vi "Test Run Suite of Several Suites.vi"(8 "error in (no error)":errorcluster, 11 "Test Case In":refnum<class "LUnit Test Suite Tests.lvclass">) -> (0 "error out":errorcluster, 3 "Test Case Out":refnum<class "LUnit Test Suite Tests.lvclass">)   [LabVIEW 2020, in "LUnit Test Suite Tests.lvclass"]
uses:
  LUnit Test Suite Tests.lvclass
  C:/Program Files (x86)/National Instruments/LabVIEW 2020/vi.lib/Astemes/LUnit/Test Case.lvclass
  source/API/LUnit Test Suite/LUnit Test Suite.lvclass
  C:/git/astemes-lunit/source/Core/Runnable/Runnable.lvclass
  Test Case Test Double/Test Case Test Double.lvclass
  C:/git/astemes-lunit/source/Core/LUnit Test Case/LUnit Test Case.lvclass
  <vilib>/Astemes/LUnit/Test Case.lvclass/Test Case.ctl
  b74e4934-f044-4222-b3dd-fc90e6c1bd4f.vi
  <vilib>/Astemes/LUnit/Palette/Pass.vi
  <vilib>/Astemes/LUnit/Palette/Fail.vi
  <vilib>/Astemes/LUnit/Compare Variants.vi
  <vilib>/Astemes/LUnit/Describe Comparison.vi
  <vilib>/Astemes/LUnit/Set Assertion Type.vi
  <vilib>/Astemes/LUnit/Add test result.vi
  <vilib>/Astemes/LUnit/Variant to string.vi
  <vilib>/Astemes/LUnit/LUnit Record Assertion Result.vi
  <vilib>/Astemes/LUnit/LUnit Aggregate Assertion Results.vi
  <vilib>/Astemes/LUnit/Method Result/LUnit Merge Status.vi
  <vilib>/Astemes/LUnit/LUnit Concatenate result strings.vi
  <vilib>/Utility/Data Type/Get Type Information.vi
  <vilib>/Utility/LVClass/Get LV Class Name.vi
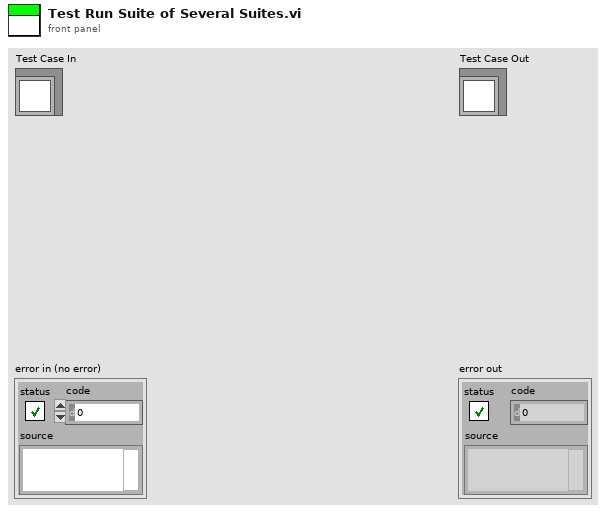
[diagram p1: front panel]
types:
  T1 = typedef "Result.lvlib/Result.ctl" = cluster{"Name":string, "Message":string, "Description":string, "Status":T2, "Result Type":T3, "Execution Time":dbl}
  T2 = typedef "Result.lvlib/Status.ctl" = enum16{"", "Passed", "Failed", "Error", "Skipped", "Setup Error", "Broken", "Teardown Error"}
  T3 = typedef "Result.lvlib/Type.ctl" = enum16{"Method", "Case", "Suite", "Pass", "Fail", "Skip", "Pass if", "Fail if", "Pass if Error", "Fail if Error", "Pass if Equal", "Fail if Equal"}
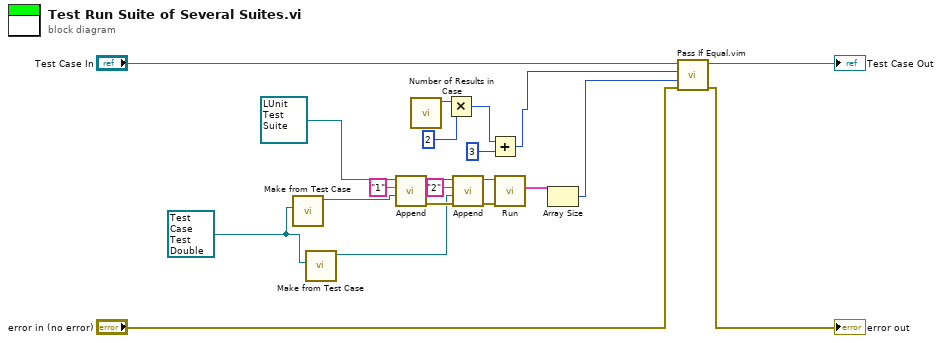
[diagram p0: block diagram]
diagram:
  w10 = refnum<class "Test Case Test Double.lvclass"> refnum ("LUnit Test Case V2 out")
  n1 = call "Make from Test Case.vi"("LUnit Test Case"=w10) -> ("LUnit Test Suite Out"=w9:refnum<class "LUnit Test Suite.lvclass">)  [unwired: 9 in, 1 out]
  n2 = call "Make from Test Case.vi"("LUnit Test Case"=w10) -> ("LUnit Test Suite Out"=w8:refnum<class "LUnit Test Suite.lvclass">)  [unwired: 9 in, 1 out]
  n3 = call "Append.vi"("Runnable"=w9, "Name"="1", "LUnit Test Suite In"=refnum<class "LUnit Test Suite.lvclass"> refnum ("LUnit Test Suite V2 in")) -> ("error out"=w13:errorcluster, "LUnit Test Suite Out"=w12:refnum<class "LUnit Test Suite.lvclass">)  [unwired: 7 in]
  n4 = call "Number of Results in Case.vi"() -> ("Number of Results"=w4:i32)  [unwired: 11 in]
  n5 = Multiply(x=w4, y=2) -> (x*y=w2:i32)
  n6 = call "Append.vi"("error in (no error)"=w13, "Runnable"=w8, "Name"="2", "LUnit Test Suite In"=w12) -> ("error out"=w15:errorcluster, "LUnit Test Suite Out"=w14:refnum<class "LUnit Test Suite.lvclass">)  [unwired: 6 in]
  n7 = Add(x=w2, y=3 ("size(s)")) -> (x+y=w3:i32)
  n8 = call-dynamic "Run.vi"("error in (no error)"=w15, "LUnit Test Suite In"=w14) -> ("Results"=w17:T1[])  [unwired: 8 in, 1 out]
  n9 = Array Size(array=w17) -> (size(s)=w16:i32)
  n10 = call "Pass If Equal.vim"("error in (no error)"="error in (no error)", "Actual"=w16, "Expected"=w3, "LUnit Test Case In"="Test Case In") -> ("error out"=→"error out":errorcluster, "LUnit Test Case Out"=→"Test Case Out":refnum<class "LUnit Test Suite Tests.lvclass">)  [unwired: 6 in]
